vi "Automatic Target Approach.vi"(0 "Main Interface":T1, 1 "Focus and Tracking":T5, 2 "System of Reference Interface":T2, 3 "Guided Approach Calibration":T7, 4 "Approach Target Button":refnum<vi>, 5 "Target":T4, 9 "Tip":T3, 11 "Error In":errorcluster, 12 "Manipulator Interface":T8, 14 "Calibration":T6) -> (15 "Error Out":errorcluster)   [LabVIEW 2012, in "Targeting Unit.lvlib"]
uses:
  Targeting Unit.lvlib
  <vilib>/Analysis/Matrix/Datatypes/RealMatrix.ctl
  <vilib>/Analysis/Matrix/NI_Matrix.lvlib
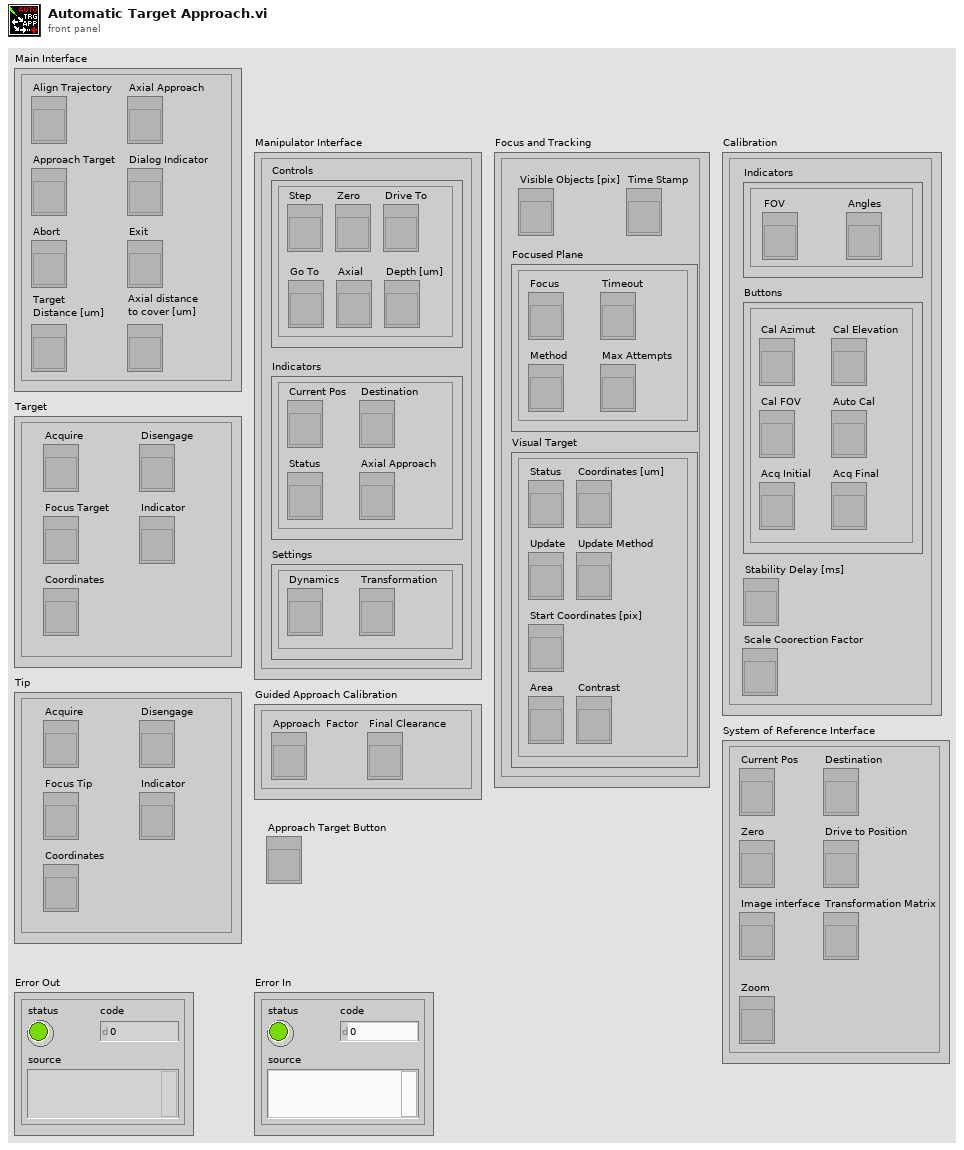
[diagram p1: front panel]
types:
  T1 = cluster{"Exit":refnum<vi>, "Abort":refnum<vi>, "Align Trajectory":refnum<vi>, "Axial Approach":refnum<vi>, "Dialog Indicator":refnum<vi>, "Approach Target":refnum<vi>, "Target\nDistance [um]":refnum<vi>, "Axial distance \nto cover [um]":refnum<vi>}
  T2 = cluster{"Current Pos":refnum<vi>, "Image interface":refnum<vi>, "Transformation Matrix":refnum<vi>, "Zero":refnum<vi>, "Destination":refnum<vi>, "Drive to Position":refnum<vi>, "Zoom":refnum<vi>}
  T3 = cluster{"Coordinates":refnum<vi>, "Acquire":refnum<vi>, "Disengage":refnum<vi>, "Indicator":refnum<vi>, "Focus Tip":refnum<vi>}
  T4 = cluster{"Coordinates":refnum<vi>, "Acquire":refnum<vi>, "Disengage":refnum<vi>, "Indicator":refnum<vi>, "Focus Target":refnum<vi>}
  T5 = cluster{"Focused Plane":cluster{"Focus":refnum<vi>, "Timeout":refnum<vi>, "Max Attempts":refnum<vi>, "Method":refnum<vi>}, "Time Stamp":refnum<vi>, "Visual Target":cluster{"Coordinates [um]":refnum<vi>, "Status":refnum<vi>, "Update":refnum<vi>, "Update Method":refnum<vi>, "Start Coordinates [pix]":refnum<vi>, "Area":refnum<vi>, "Contrast":refnum<vi>}, "Visible Objects [pix]":refnum<vi>}
  T6 = cluster{"Indicators":cluster{"FOV":refnum<vi>, "Angles":refnum<vi>}, "Buttons":cluster{"Cal FOV":refnum<vi>, "Cal Azimut":refnum<vi>, "Cal Elevation":refnum<vi>, "Auto Cal":refnum<vi>, "Acq Initial":refnum<vi>, "Acq Final":refnum<vi>}, "Stability Delay [ms]":refnum<vi>, "Scale Coorection Factor":refnum<vi>}
  T7 = cluster{"Approach  Factor":refnum<vi>, "Final Clearance":refnum<vi>}
  T8 = cluster{"Indicators":cluster{"Current Pos":refnum<vi>, "Destination":refnum<vi>, "Status":refnum<vi>, "Axial Approach":refnum<vi>}, "Settings":cluster{"Dynamics":refnum<vi>, "Transformation":refnum<vi>}, "Controls":cluster{"Zero":refnum<vi>, "Step":refnum<vi>, "Drive To":refnum<vi>, "Go To":refnum<vi>, "Axial":refnum<vi>, "Depth [um]":refnum<vi>}}
  T9 = cluster{"X [um]":dbl, "Y [um]":dbl, "Z [um]":dbl}
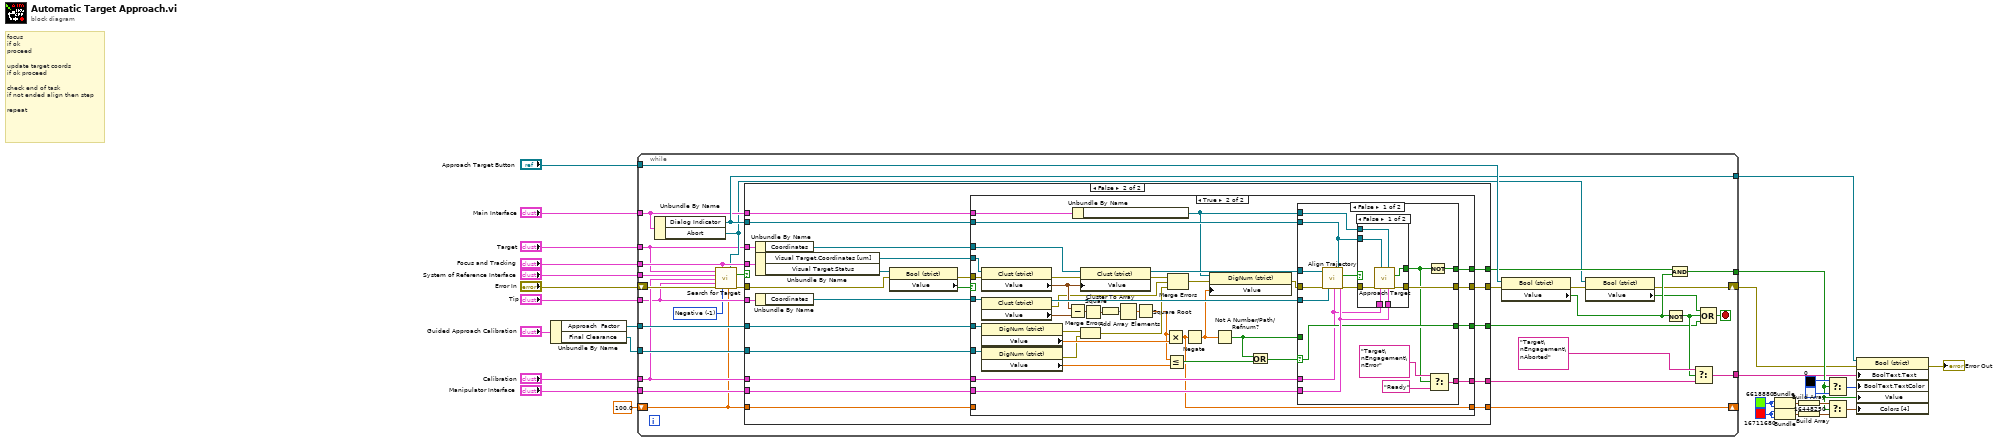
[diagram p0: block diagram]
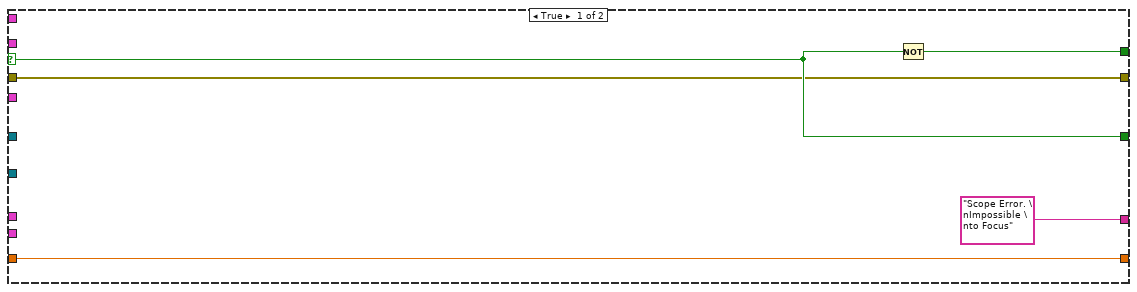
[diagram p2: hidden frame]
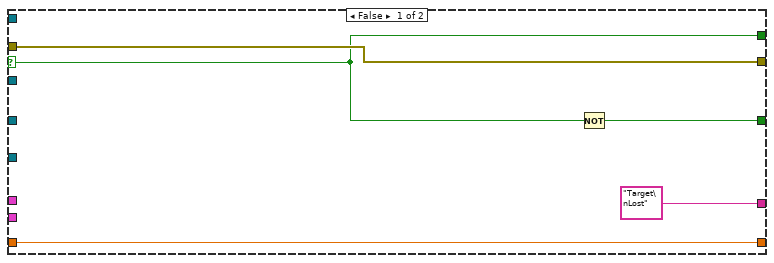
[diagram p3: hidden frame]
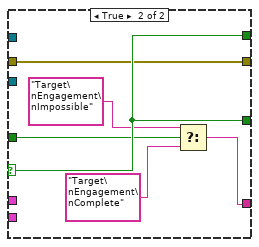
[diagram p5: hidden frame]
diagram:
  w9 = u32 16711680
  w12 = u32 6618880
  # "focus\nif ok\nproceed\n\nupdate target coords\nif ok proceed\n\ncheck end of task\nif not ended align then step\n\nrepeat"
  n1 = Unbundle By Name("Guided Approach Calibration") -> ("Approach  Factor"=w17:refnum<vi>, "Final Clearance"=w16:refnum<vi>)
  n2 = while {
    tunnel: "Manipulator Interface" -> [w58]
    tunnel: "Calibration" -> [w46]
    shift-right: [w39] -> w3
    shift-left: "Error In" -> [w48]
    tunnel: w17 -> [w57]
    tunnel: w16 -> [w59]
    tunnel: "Focus and Tracking" -> [w42]
    tunnel: [w50] -> w5
    tunnel: [w56] -> w4
    tunnel: "Approach Target Button" -> [w54]
    tunnel: "Target" -> [w33]
    tunnel: "Tip" -> [w32]
    tunnel: "System of Reference Interface" -> [w45]
    tunnel: "Main Interface" -> [w41]
    tunnel: [w43] -> w2
    shift-right: [w31] -> _
    shift-left: 100.0 -> [w30]
    stop <- w37 stop-if-true
    w29 = i8 -1 items=["Positive"=1, "Negative"=-1] ("Z direction")
    n3 = Unbundle By Name(w41) -> ("Dialog Indicator"=w43:refnum<vi>, "Abort"=w34:refnum<vi>)
    n4 = call "Search for Target.vi"("Target"=w33, "Focus and Tracking"=w42, "Calibration"=w46, "Tip"=w32, "Max Distance [um]"=w30, "Error In"=w48, "System of Reference Interface"=w45, "Z direction"=w29, "Abort"=w34) -> ("Scope Error"=w44:bool, "Error Out"=w47:errorcluster)  [unwired: 4 in, 1 out]
    n5 = case shown="False" w44 {
      selector: w44 -> [w63 _]
      tunnel: w47 -> [w61 w71]
      tunnel: [w63 w84] -> w36
      tunnel: ["Scope Error. \nImpossible \nto Focus" ("f") w83] -> w53
      tunnel: w59 -> [_ w82]
      tunnel: w33 -> [_ w68]
      tunnel: w32 -> [_ w70]
      tunnel: w58 -> [_ w81]
      tunnel: w46 -> [_ w80]
      tunnel: w57 -> [_ w79]
      tunnel: [w62 w78] -> w51
      tunnel: [w61 w77] -> w55
      tunnel: w42 -> [_ w74]
      tunnel: w41 -> [_ w73]
      tunnel: w43 -> [_ w72]
      tunnel: [w60 w66] -> w31
      tunnel: w30 -> [w60 w65]
      frame True {
        n6 = Not(x=w63) -> (.not. x?=w62:bool)
      }
      frame False {
        n7 = Unbundle By Name(w68) -> ("Coordinates"=w67:refnum<vi>)
        n8 = Unbundle By Name(w74) -> ("Visual Target.Coordinates [um]"=w76:refnum<vi>, "Visual Target.Status"=w75:refnum<vi>)
        n9 = Unbundle By Name(w70) -> ("Coordinates"=w69:refnum<vi>)
        n10 = property class="Bool (strict)"(reference=w75, error in=w71) -> (error out=w86:errorcluster, "Value"=w85:bool)  [unwired: 1 out]
        n11 = case shown="True" w85 {
          selector: w85 -> [w88 _]
          tunnel: w76 -> [_ w130]
          tunnel: w86 -> [w91 w103]
          tunnel: [w91 w119] -> w77
          tunnel: [w89 w120] -> w84
          tunnel: ["Target\nLost" ("f") w121] -> w83
          tunnel: w82 -> [_ w122]
          tunnel: w67 -> [_ w94]
          tunnel: w81 -> [_ w118]
          tunnel: w80 -> [_ w117]
          tunnel: w79 -> [_ w108]
          tunnel: [w88 w115] -> w78
          tunnel: w73 -> [_ w110]
          tunnel: w72 -> [_ w109]
          tunnel: w69 -> [_ w95]
          tunnel: [w87 w92] -> w66
          tunnel: w65 -> [w87 _]
          frame False {
            n12 = Not(x=w88) -> (.not. x?=w89:bool)
          }
          frame True {
            n13 = property class="DigNum (strict)"(reference=w108) -> (error out=w101:errorcluster, "Value"=w107:dbl)  [unwired: 1 in, 1 out]
            n14 = property class="DigNum (strict)"(reference=w122) -> (error out=w102:errorcluster, "Value"=w127:dbl)  [unwired: 1 in, 1 out]
            n15 = property class="Clust (strict)"(reference=w130, error in=w103) -> (error out=w129:errorcluster, "Value"=w113:cluster{"X":dbl, "Y":dbl, "Z":dbl})  [unwired: 1 out]
            n16 = property class="Clust (strict)"(reference=w95) -> (reference out=w116:refnum<vi>, error out=w112:errorcluster, "Value"=w128:T9)  [unwired: 1 in]
            n17 = Subtract(x=w113, y=w128) -> (x-y=w126:cluster{dbl, dbl, dbl})
            n18 = Unbundle By Name(w110) -> ("Axial distance \nto cover [um]"=w104:refnum<vi>)
            n19 = property class="Clust (strict)"(reference=w94, error in=w129, "Value"=w113) -> (reference out=w114:refnum<vi>, error out=w111:errorcluster)
            n20 = Merge Errors(w101, w102) -> (w100:errorcluster)
            n21 = Square(x=w126) -> (x^2=w123:cluster{dbl, dbl, dbl})
            n22 = Cluster To Array(cluster=w123) -> (array=w124:dbl[])
            n23 = Add Array Elements(numeric array=w124) -> (sum=w125:dbl)
            n24 = Square Root(x=w125) -> (sqrt(x)=w93:dbl)
            n25 = Multiply(x=w93, y=w107) -> (x*y=w92:dbl)
            n26 = Less Or Equal?(x=w93, y=w127) -> (x <= y?=w99:bool)
            n27 = Merge Errors(w111, w112, w100) -> (w106:errorcluster)
            n28 = Negate(x=w92) -> (-x=w96:dbl)
            n29 = property class="DigNum (strict)"(reference=w104, error in=w106, "Value"=w96) -> (error out=w105:errorcluster)  [unwired: 1 out]
            n30 = Not A Number/Path/Refnum?(number/path/refnum=w96) -> (NaN/Path/Refnum?=w97:bool)
            n31 = Or(x=w97, y=w99) -> (x .or. y?=w98:bool)
            n32 = case shown="False" w98 {
              selector: w98 -> [w135 w161]
              tunnel: [w138 w159] -> w121
              tunnel: [w135 w161] -> w120
              tunnel: [w144 w160] -> w119
              tunnel: w118 -> [w136 _]
              tunnel: w109 -> [w141 _]
              tunnel: w117 -> [w132 _]
              tunnel: w114 -> [w142 _]
              tunnel: w116 -> [w143 _]
              tunnel: w105 -> [w140 w160]
              tunnel: [w133 w161] -> w115
              tunnel: w104 -> [w131 _]
              tunnel: w97 -> [_ w157]
              frame False {
                n33 = call "Align Trajectory.vi"("Indicator"=w141, "Calibration"=w132, "error in"=w140, "Tip Coordinates"=w143, "Target Coordinates"=w142, "Manipulator Interface"=w136) -> ("error out"=w145:errorcluster, "Error"=w146:bool)  [unwired: 4 in]
                n34 = case shown="False" w146 {
                  selector: w146 -> [_ w154]
                  tunnel: w145 -> [w153 w155]
                  tunnel: w136 -> [w152 _]
                  tunnel: [w151 w155] -> w144
                  tunnel: w141 -> [w149 _]
                  tunnel: [w150 w154] -> w134
                  tunnel: w132 -> [w148 _]
                  tunnel: w131 -> [w147 _]
                  frame False {
                    n35 = call "Approach Target.vi"("Indicator"=w149, "Axial distance [um]"=w147, "error in"=w153, "Calibration"=w148, "Manipulator Interface"=w152) -> ("error out"=w151:errorcluster, "Error"=w150:bool)  [unwired: 5 in]
                  }
                  frame True {
                  }
                }
                n36 = Not(x=w134) -> (.not. x?=w133:bool)
                n37 = Select(t="Target\nEngagement\nError", s=w134, f="Ready" ("t")) -> (s? t:f=w138:string)
              }
              frame True {
                n38 = Select(t="Target\nEngagement\nImpossible", s=w157, f="Target\nEngagement\nComplete" ("t")) -> (s? t:f=w159:string)
              }
            }
          }
        }
      }
    }
    n39 = property class="Bool (strict)"(reference=w54, error in=w55) -> (error out=w40:errorcluster, "Value"=w49:bool)  [unwired: 1 out]
    n40 = property class="Bool (strict)"(reference=w34, error in=w40) -> (error out=w39:errorcluster, "Value"=w35:bool)  [unwired: 1 out]
    n41 = Not(x=w49) -> (.not. x?=w38:bool)
    n42 = And(x=w51, y=w49) -> (x .and. y?=w50:bool)
    n43 = Select(t="Target\nEngagement\nAborted", s=w38, f=w53) -> (s? t:f=w56:string)
    n44 = Compound Arithmetic op=OR(w35, w38, w36) -> (w37:bool)
  }
  n45 = Bundle(w12, w12) -> (w11:cluster{u32, u32})  [unwired: 1 in]
  n46 = Bundle(w9, w9) -> (w8:cluster{u32, u32})  [unwired: 1 in]
  n47 = Build Array(w11) -> (w10:cluster{u32, u32}[])
  n48 = Build Array(w8) -> (w7:cluster{u32, u32}[])
  n49 = Select(t=u32 0, s=w5, f=u32 16448250) -> (s? t:f=w13:u32)
  n50 = Select(t=w10, s=w5, f=w7) -> (s? t:f=w6:cluster{u32, u32}[])
  n51 = property class="Bool (strict)"(reference=w2, error in=w3, "BoolText.Text"=w4, "BoolText.TextColor"=w13, "Value"=w5, "Colors [4]"=w6) -> (error out=→"Error Out":errorcluster)  [unwired: 1 out]
